vi "test Initialize Clear Count.vi"(8 "error in (no error)":errorcluster, 11 "TestCase in":refnum<class "Channel Manager.lvclass">) -> (0 "error out":errorcluster, 3 "TestCase out":refnum<class "Channel Manager.lvclass">)   [LabVIEW 2020, in "Channel Manager.lvclass"]
uses:
  Channel Manager.lvclass
  Hardware API/Channel Status.ctl
  Hardware API/Channel Action.ctl
  <vilib>/addons/_JKI Toolkits/VI Tester/TestCase.llb/TestCase.lvclass
  Hardware API/AIM ARINC 429 Hardware API.lvlib
  C:/Program Files (x86)/National Instruments/LabVIEW 2020/vi.lib/addons/_JKI Toolkits/VI Tester/TestCase.llb/TestCase.lvclass
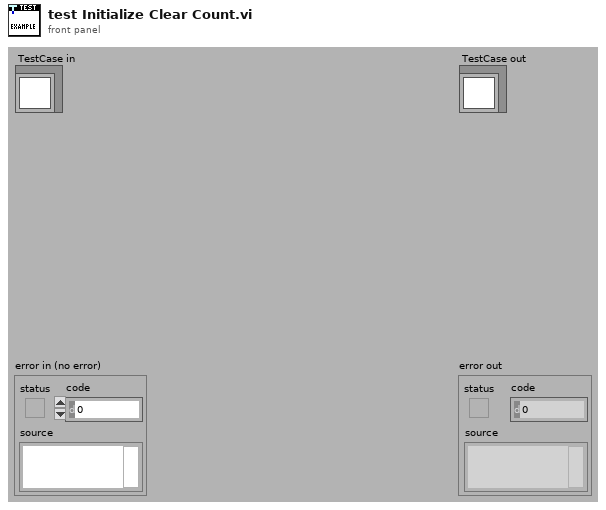
[diagram p1: front panel]
types:
  T1 = typedef "AIM ARINC 429 Hardware API.lvlib/Channel Action.ctl" = enum16{"Get Info", "Initialize", "Start", "Clear"}
  T2 = typedef "AIM ARINC 429 Hardware API.lvlib/Channel Status.ctl" = enum16{"Uninitialized", "Idle", "Active"}
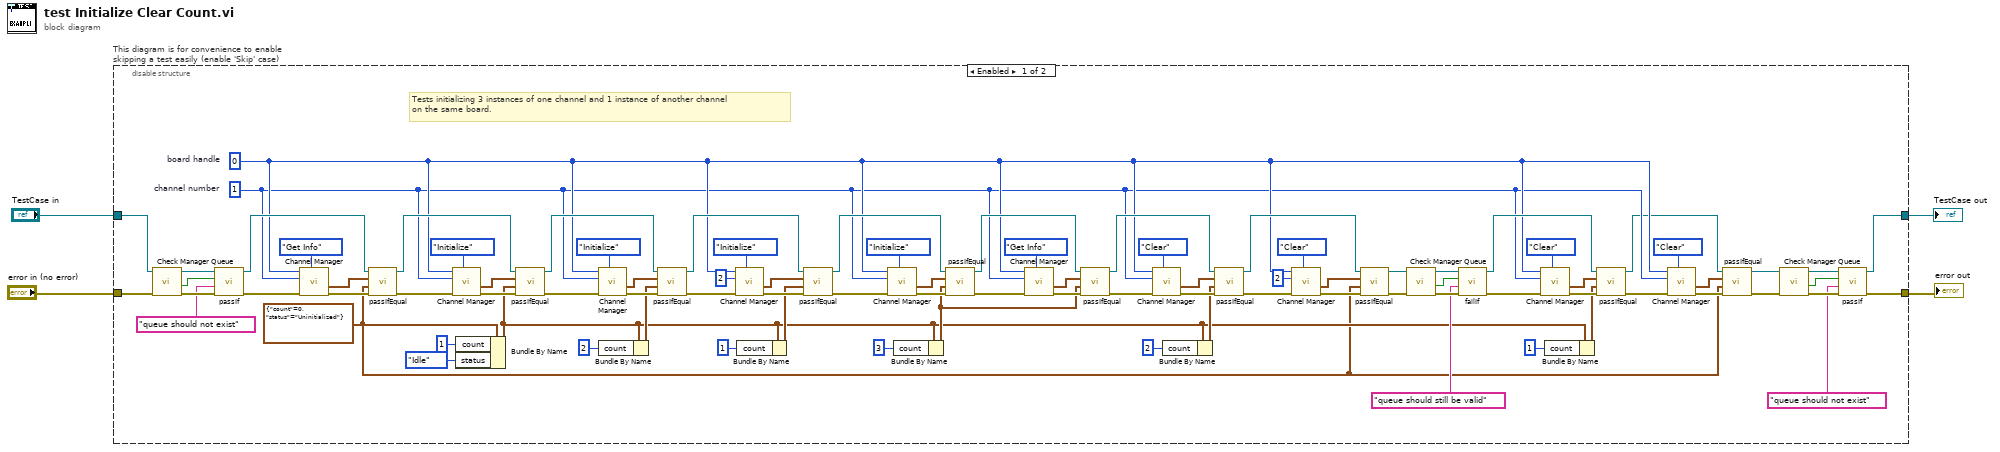
[diagram p0: block diagram]
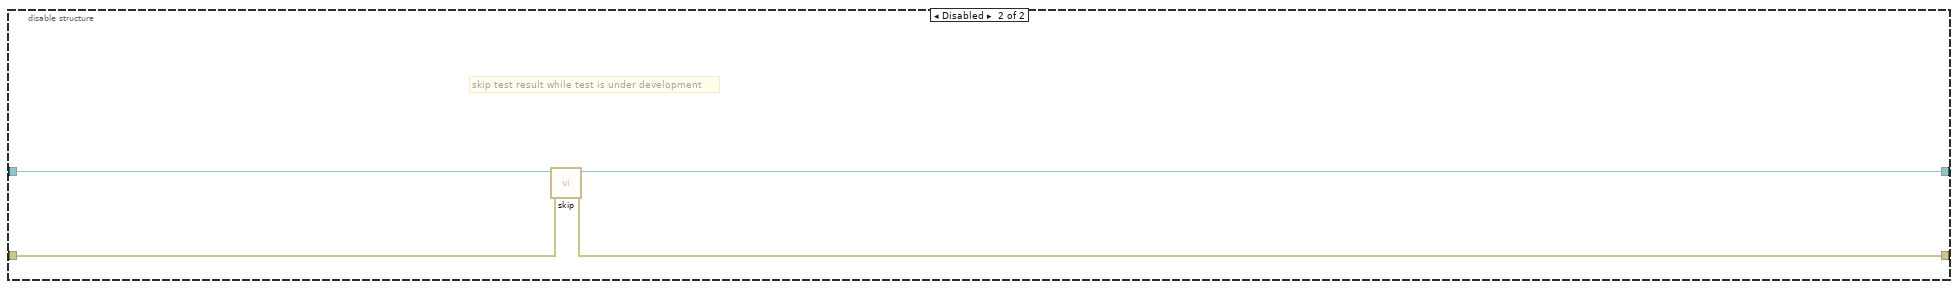
[diagram p2: hidden frame]
diagram:
  n1 = disable-structure "This diagram is for convenience to enable skipping a test easily (enable 'Skip' case)" shown="Enabled" {
    disable-tunnel: "TestCase in" -> [w83 w96]
    disable-tunnel: [w8 w94] -> w1
    disable-tunnel: [w7 w95] -> w3
    disable-tunnel: "error in (no error)" -> [w92 w93]
    frame Enabled {
      w13 = cluster{"count":u32, "status":T2} {"count"=0, "status"=enum."Uninitialized"} ("channel info")
      w17 = u8 1  # channel number
      w18 = u8 0  # board handle
      # "Tests initializing 3 instances of one channel and 1 instance of another channel\non the same board."
      n2 = call "Check Manager Queue.vi"("error in (no error)"=w92, "Channel Manager in"=w83) -> ("error out"=w91:errorcluster, "queue ref invalid"=w89:bool, "Channel Manager out"=w90:refnum<class "Channel Manager.lvclass">)  [unwired: 7 in]
      n3 = call-dynamic "passIf.vi"("error in (no error)"=w91, "message (\"\")"="queue should not exist" ("message (\"\")"), "pass"=w89, "TestCase in"=w90) -> ("error out"=w87:errorcluster, "TestCase out"=w80:refnum<class "Channel Manager.lvclass">)  [unwired: 6 in]
      n4 = call "Channel Manager.vi"("action"=Channel_Action."Get Info", "error in"=w87, "channel number"=w17, "board handle"=w18) -> ("error out"=w85:errorcluster, "channel info"=w84:cluster{"count":u32, "status":T2})  [unwired: 4 in, 2 out]
      n5 = call-dynamic "passIfEqual.vi"("error in (no error)"=w85, "y"=w13, "x"=w84, "TestCase in"=w80) -> ("error out"=w81:errorcluster, "TestCase out"=w79:refnum<class "Channel Manager.lvclass">)  [unwired: 6 in]
      n6 = call "Channel Manager.vi"("action"=Channel_Action."Initialize", "error in"=w81, "channel number"=w17, "board handle"=w18) -> ("error out"=w78:errorcluster, "channel info"=w77:cluster{"count":u32, "status":T2})  [unwired: 4 in, 2 out]
      n7 = Bundle By Name(cluster=w13, "count"=u32 1, "status"=Channel_Status."Idle") -> (w25:cluster{"count":u32, "status":T2})
      n8 = call-dynamic "passIfEqual.vi"("error in (no error)"=w78, "y"=w25, "x"=w77, "TestCase in"=w79) -> ("error out"=w73:errorcluster, "TestCase out"=w65:refnum<class "Channel Manager.lvclass">)  [unwired: 6 in]
      n9 = call "Channel Manager.vi"("action"=Channel_Action."Initialize", "error in"=w73, "channel number"=w17, "board handle"=w18) -> ("error out"=w71:errorcluster, "channel info"=w72:cluster{"count":u32, "status":T2})  [unwired: 4 in, 2 out]
      n10 = Bundle By Name(cluster=w25, "count"=u32 2) -> (w69:cluster{"count":u32, "status":T2})
      n11 = call-dynamic "passIfEqual.vi"("error in (no error)"=w71, "y"=w69, "x"=w72, "TestCase in"=w65) -> ("error out"=w67:errorcluster, "TestCase out"=w63:refnum<class "Channel Manager.lvclass">)  [unwired: 6 in]
      n12 = call "Channel Manager.vi"("action"=Channel_Action."Initialize", "error in"=w67, "channel number"=u8 2, "board handle"=w18) -> ("error out"=w64:errorcluster, "channel info"=w62:cluster{"count":u32, "status":T2})  [unwired: 4 in, 2 out]
      n13 = Bundle By Name(cluster=w25, "count"=u32 1) -> (w60:cluster{"count":u32, "status":T2})
      n14 = call-dynamic "passIfEqual.vi"("error in (no error)"=w64, "y"=w60, "x"=w62, "TestCase in"=w63) -> ("error out"=w58:errorcluster, "TestCase out"=w55:refnum<class "Channel Manager.lvclass">)  [unwired: 6 in]
      n15 = call "Channel Manager.vi"("action"=Channel_Action."Initialize", "error in"=w58, "channel number"=w17, "board handle"=w18) -> ("error out"=w56:errorcluster, "channel info"=w54:cluster{"count":u32, "status":T2})  [unwired: 4 in, 2 out]
      n16 = Bundle By Name(cluster=w25, "count"=u32 3) -> (w45:cluster{"count":u32, "status":T2})
      n17 = call-dynamic "passIfEqual.vi"("error in (no error)"=w56, "y"=w45, "x"=w54, "TestCase in"=w55) -> ("error out"=w52:errorcluster, "TestCase out"=w50:refnum<class "Channel Manager.lvclass">)  [unwired: 6 in]
      n18 = call "Channel Manager.vi"("action"=Channel_Action."Get Info", "error in"=w52, "channel number"=w17, "board handle"=w18) -> ("error out"=w51:errorcluster, "channel info"=w49:cluster{"count":u32, "status":T2})  [unwired: 4 in, 2 out]
      n19 = call-dynamic "passIfEqual.vi"("error in (no error)"=w51, "y"=w45, "x"=w49, "TestCase in"=w50) -> ("error out"=w47:errorcluster, "TestCase out"=w43:refnum<class "Channel Manager.lvclass">)  [unwired: 6 in]
      n20 = call "Channel Manager.vi"("action"=Channel_Action."Clear", "error in"=w47, "channel number"=w17, "board handle"=w18) -> ("error out"=w44:errorcluster, "channel info"=w41:cluster{"count":u32, "status":T2})  [unwired: 4 in, 2 out]
      n21 = Bundle By Name(cluster=w25, "count"=u32 2) -> (w42:cluster{"count":u32, "status":T2})
      n22 = call-dynamic "passIfEqual.vi"("error in (no error)"=w44, "y"=w42, "x"=w41, "TestCase in"=w43) -> ("error out"=w39:errorcluster, "TestCase out"=w37:refnum<class "Channel Manager.lvclass">)  [unwired: 6 in]
      n23 = call "Channel Manager.vi"("action"=Channel_Action."Clear", "error in"=w39, "channel number"=u8 2, "board handle"=w18) -> ("error out"=w36:errorcluster, "channel info"=w35:cluster{"count":u32, "status":T2})  [unwired: 4 in, 2 out]
      n24 = call-dynamic "passIfEqual.vi"("error in (no error)"=w36, "y"=w13, "x"=w35, "TestCase in"=w37) -> ("error out"=w33:errorcluster, "TestCase out"=w34:refnum<class "Channel Manager.lvclass">)  [unwired: 6 in]
      n25 = call "Check Manager Queue.vi"("error in (no error)"=w33, "Channel Manager in"=w34) -> ("error out"=w32:errorcluster, "queue ref invalid"=w30:bool, "Channel Manager out"=w31:refnum<class "Channel Manager.lvclass">)  [unwired: 7 in]
      n26 = call-dynamic "failIf.vi"("error in (no error)"=w32, "message (\"\")"="queue should still be valid" ("message (\"\")"), "fail"=w30, "TestCase in"=w31) -> ("error out"=w27:errorcluster, "TestCase out"=w23:refnum<class "Channel Manager.lvclass">)  [unwired: 6 in]
      n27 = call "Channel Manager.vi"("action"=Channel_Action."Clear", "error in"=w27, "channel number"=w17, "board handle"=w18) -> ("error out"=w24:errorcluster, "channel info"=w21:cluster{"count":u32, "status":T2})  [unwired: 4 in, 2 out]
      n28 = Bundle By Name(cluster=w25, "count"=u32 1) -> (w22:cluster{"count":u32, "status":T2})
      n29 = call-dynamic "passIfEqual.vi"("error in (no error)"=w24, "y"=w22, "x"=w21, "TestCase in"=w23) -> ("error out"=w19:errorcluster, "TestCase out"=w15:refnum<class "Channel Manager.lvclass">)  [unwired: 6 in]
      n30 = call "Channel Manager.vi"("action"=Channel_Action."Clear", "error in"=w19, "channel number"=w17, "board handle"=w18) -> ("error out"=w16:errorcluster, "channel info"=w14:cluster{"count":u32, "status":T2})  [unwired: 4 in, 2 out]
      n31 = call-dynamic "passIfEqual.vi"("error in (no error)"=w16, "y"=w13, "x"=w14, "TestCase in"=w15) -> ("error out"=w12:errorcluster, "TestCase out"=w11:refnum<class "Channel Manager.lvclass">)  [unwired: 6 in]
      n32 = call "Check Manager Queue.vi"("error in (no error)"=w12, "Channel Manager in"=w11) -> ("error out"=w10:errorcluster, "queue ref invalid"=w6:bool, "Channel Manager out"=w9:refnum<class "Channel Manager.lvclass">)  [unwired: 7 in]
      n33 = call-dynamic "passIf.vi"("error in (no error)"=w10, "message (\"\")"="queue should not exist" ("message (\"\")"), "pass"=w6, "TestCase in"=w9) -> ("error out"=w7:errorcluster, "TestCase out"=w8:refnum<class "Channel Manager.lvclass">)  [unwired: 6 in]
    }
    frame Disabled {
      # "skip test result while test is under development"
      n34 = call <vilib>:"skip.vi"("error in (no error)"=w93, "TestCase in"=w96) -> ("error out"=w95:errorcluster, "TestCase out"=w94:refnum<class "Channel Manager.lvclass">)  [unwired: 8 in]
    }
  }
  "error out" <- w3
  "TestCase out" <- w1
